vi "Launcher (top level).vi"   [LabVIEW 2021]
uses:
  Utils/AF Utils.lvlib
  Actors/Game/Game/Game.lvclass
  C:/Program Files (x86)/National Instruments/LabVIEW 2021/vi.lib/ActorFramework/Actor/Actor.lvclass
  C:/Repositories/LabVIEW/Actor/Actor-Dice-Game/src/Actors/Game/Game/Game.lvclass
panel:
  # "This is a top level VI for this Project.  When it runs it will spawn a\nloading screen and then open the actor for the project to run."
  # "James Sizeland, 2022"
types:
  T1 = enum32{"Invalid", "Standard", "Closed", "Hidden", "Minimized", "Maximized"}
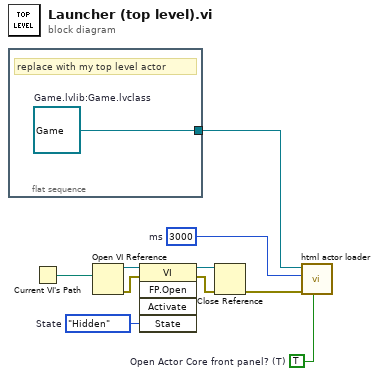
[diagram p0: block diagram]
diagram:
  w4 = T1."Hidden"  # State
  w8 = TRUE  # Open Actor Core front panel? (T)
  w10 = u32 3000  # ms
  n1 = flat-sequence {
    tunnel: [w11] -> w9
    frame #0 {
      w11 = refnum<class "Game.lvclass"> refnum  # Game.lvlib:Game.lvclass
      # "replace with my top level actor"
    }
  }
  n2 = Current VI's Path() -> (path=w7:path)
  n3 = Open VI Reference(vi path=w7) -> (vi reference=w6:refnum<vi>, error out=w5:errorcluster)  [unwired: 5 in]
  n4 = invoke class="VI" method="FP.Open"(reference=w6, error in=w5, "State"=w4) -> (reference out=w3:refnum<vi>, error out=w2:errorcluster)  [unwired: 2 in, 3 out]
  n5 = Close Reference(reference=w3, error in (no error)=w2) -> (error out=w1:errorcluster)
  n6 = call "html actor loader.vi"("Open Actor Core front panel? (T)"=w8, "error in (no error)"=w1, "runtime (3000ms)"=w10, "Actor"=w9) -> ()  [unwired: 7 in, 1 out]
